vi "Process.vi"(8 "error in":errorcluster, 11 "Plugin in":refnum<class "Sequencer with Output Values.lvclass">) -> (0 "error out":errorcluster, 3 "Plugin out":refnum<class "Sequencer with Output Values.lvclass">)   [LabVIEW 2024, in "Sequencer with Output Values.lvlib" / "Sequencer with Output Values.lvclass"]
uses:
  Sequencer with Output Values.lvclass
  C:/Program Files/National Instruments/LabVIEW 2024/vi.lib/FlexLogger/SDK/PluginSDK.lvlibp/PEFClasses/SDK/Plugin/Plugin.lvclass
  <vilib>/FlexLogger/SDK/PluginSDK.lvlibp/PEFClasses/SDK/Plugin/DataHelpers/Write 1D DBL (NChan 1Sample).vi
  <vilib>/FlexLogger/SDK/PluginSDK.lvlibp/PEFClasses/SDK/Plugin/DataHelpers/Write 1D Bool (NChan 1 Sample).vi
  Global Strings.vi
  <vilib>/FlexLogger/SDK/PluginSDK.lvlibp/PEFClasses/SDK/Plugin/ParameterAccess/Write String.vi
  <vilib>/FlexLogger/SDK/PluginSDK.lvlibp/PEFClasses/SDK/Plugin/Plugin.lvclass
  C:/Program Files/National Instruments/LabVIEW 2024/vi.lib/FlexLogger/SDK/PluginSDK.lvlibp/PEFClasses/SDK/Processing Element/Processing Element.lvclass
  C:/dev/niflexlogger-plugins/plugins/Sequencer with Output Values/source/Sequencer with Output Values/Sequencer with Output Values.lvclass
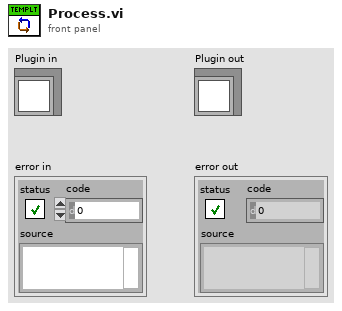
[diagram p1: front panel]
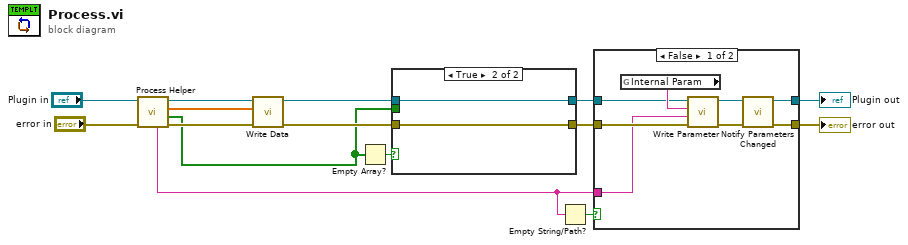
[diagram p0: block diagram]
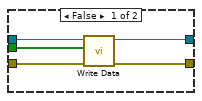
[diagram p3: hidden frame]
diagram:
  n1 = call "Process Helper.vi"("error in (no error)"="error in", "Plugin in"="Plugin in") -> ("error out"=w6:errorcluster, "Digital Values to Write"=w5:bool[], "Analog Values to Write"=w1:dbl[], "Plugin out"=w4:refnum<class "Sequencer with Output Values.lvclass">, "New Flatterned Params (Empty if no change)"=w3:string)  [unwired: 5 in]
  n2 = call-poly <vilib>:"Write Data.vi"("error in (no error)"=w6, "Data"=w1, "Plugin in"=w4) -> ("error out"=w10:errorcluster, "Plugin out"=w11:refnum<class "Sequencer with Output Values.lvclass">)  [unwired: 7 in]
  n3 = Empty Array?(array=w5) -> (empty?=w9:bool)
  n4 = case shown="True" w9 {
    tunnel: w11 -> [w20 w22]
    tunnel: w10 -> [w19 w21]
    tunnel: [w18 w22] -> w7
    tunnel: [w17 w21] -> w8
    tunnel: w5 -> [w16 _]
    frame False {
      n5 = call-poly <vilib>:"Write Data.vi"("error in (no error)"=w19, "Data"=w16, "Plugin in"=w20) -> ("error out"=w17:errorcluster, "Plugin out"=w18:refnum<class "Sequencer with Output Values.lvclass">)  [unwired: 7 in]
    }
    frame True {
    }
  }
  n6 = Empty String/Path?(string/path=w3) -> (empty?=w2:bool)
  n7 = case shown="False" w2 {
    tunnel: w8 -> [w28 w31]
    tunnel: w7 -> [w29 w32]
    tunnel: [w27 w32] -> w15
    tunnel: [w26 w31] -> w12
    tunnel: w3 -> [w25 _]
    frame False {
      n8 = global read "Global Strings.vi" "Internal Param"() -> (w30:string)
      n9 = call-poly <vilib>:"Write Parameter.vi"("error in (no error)"=w28, "Value"=w25, "Name"=w30, "Plugin in"=w29) -> ("error out"=w23:errorcluster, "Plugin out"=w24:refnum<class "Sequencer with Output Values.lvclass">)  [unwired: 6 in]
      n10 = call <vilib>:"Notify Parameters Changed.vi"("error in (no error)"=w23, "Plugin in"=w24) -> ("error out"=w26:errorcluster, "Plugin out"=w27:refnum<class "Sequencer with Output Values.lvclass">)  [unwired: 8 in]
    }
    frame True {
    }
  }
  "error out" <- w12
  "Plugin out" <- w15
